vi "Initialize.vi"(8 "error in (no error)":errorcluster, 11 "S4ACS_GUI in":refnum<class "S4GUI.lvclass">) -> (0 "error out":errorcluster, 3 "S4ACS_GUI out":refnum<class "S4GUI.lvclass">)   [LabVIEW 2018, in "S4GUI.lvclass"]
uses:
  S4GUI.lvclass
  S4GUI.lvclass/S4GUI.ctl
  Publisher/Publisher.lvclass
  GSserver/GSserver.lvclass
  WeatherStation/WeatherStation.lvclass
  TelFocus/TelFocus.lvclass
  TCS/TCS.lvclass
  Instrument/Instrument.lvclass
  Acquisition/Acquisition.lvclass
  SyncBox/Sync Box.lvclass
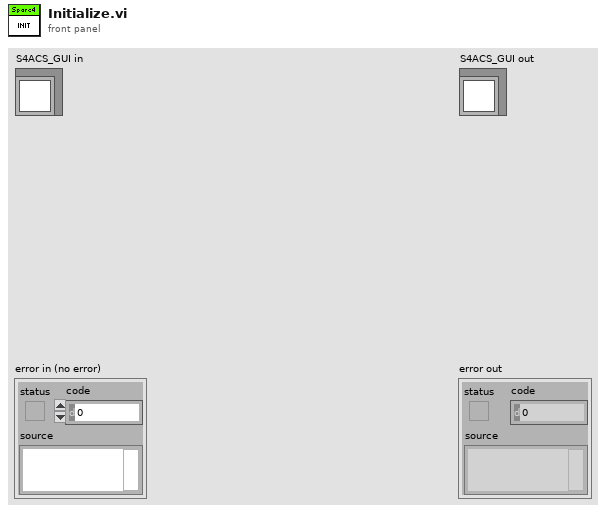
[diagram p1: front panel]
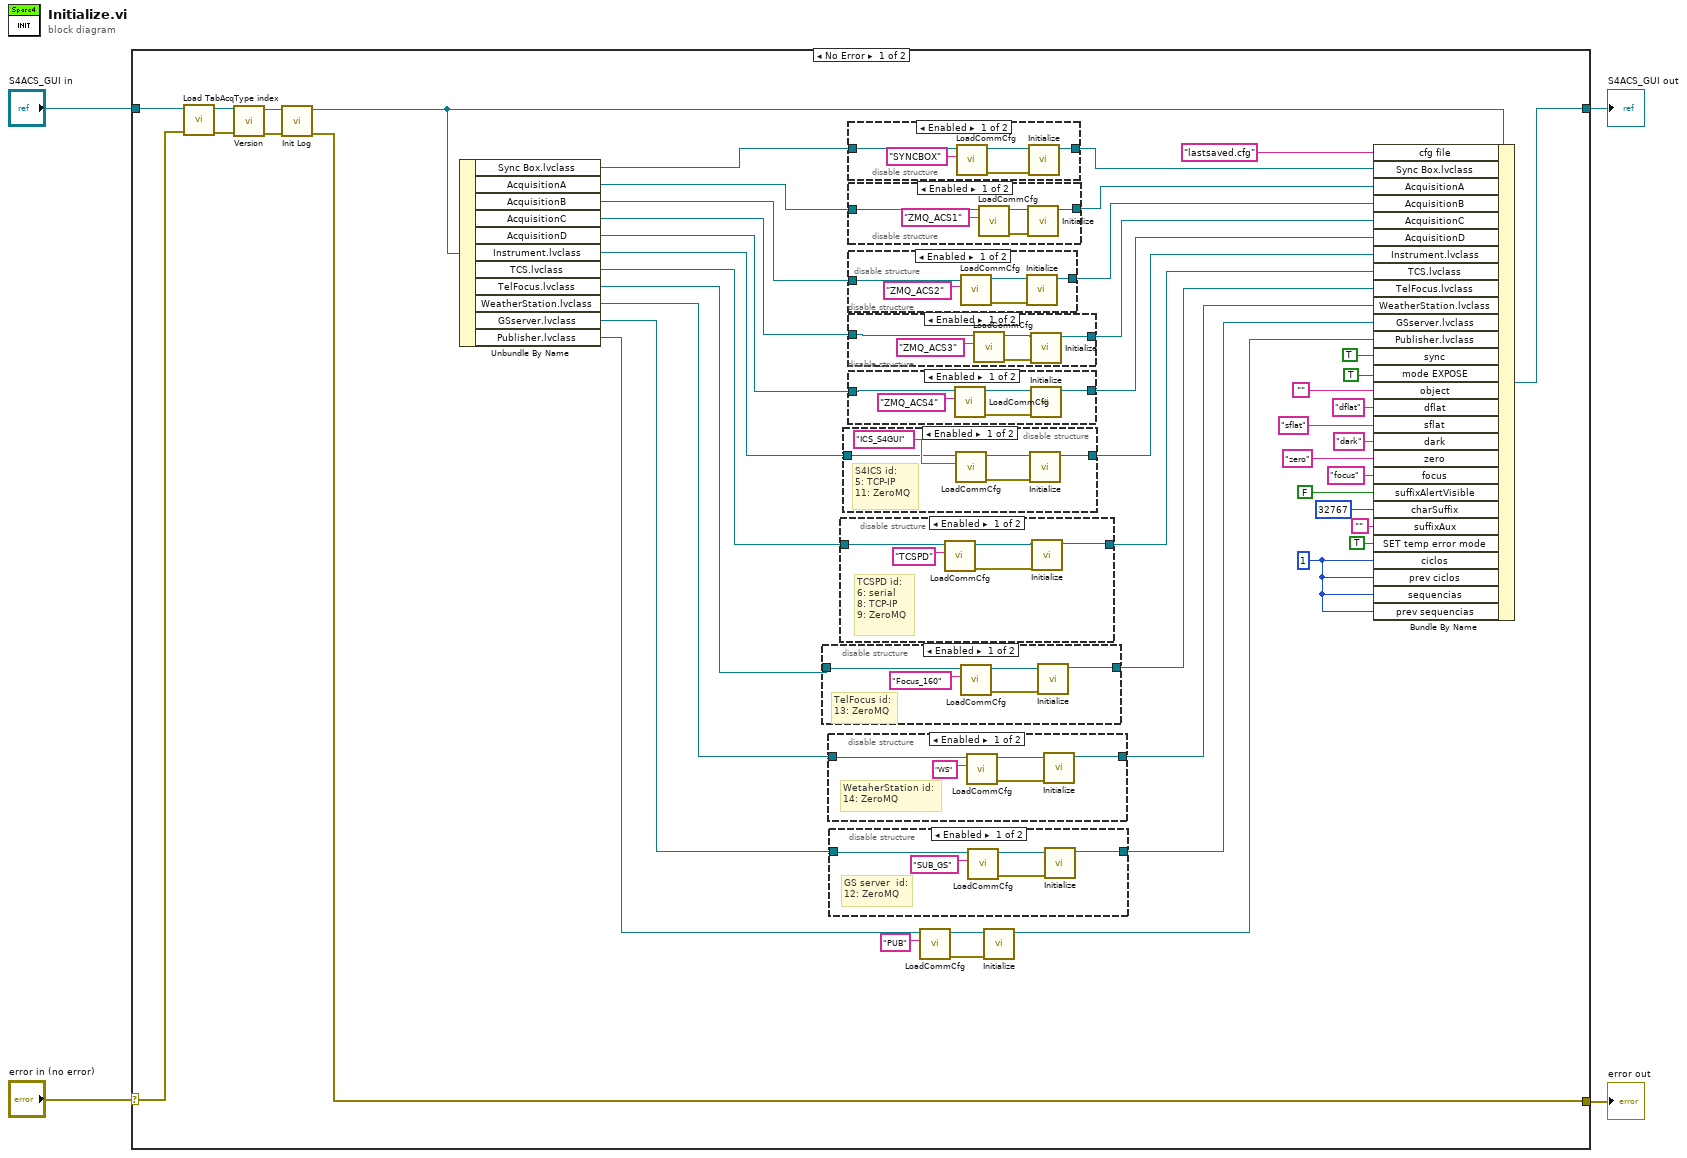
[diagram p0: block diagram]
diagram:
  n1 = case shown="No Error" "error in (no error)" {
    selector: "error in (no error)" -> [w20 w114]
    tunnel: [w23 w114] -> w3
    tunnel: [w31 w113] -> w1
    tunnel: "S4ACS_GUI in" -> [w18 w113]
    frame No Error {
      w5 = u32 1 ("ciclos")
      n2 = call-dynamic "Load TabAcqType index.vi"("error in (no error)"=w20, "S4GUI in"=w18) -> ("error out"=w19:errorcluster, "S4GUI out"=w17:refnum<class "S4GUI.lvclass">)  [unwired: 8 in]
      n3 = call-dynamic "Version.vi"("error in (no error)"=w19, "S4GUI in"=w17) -> ("error out"=w22:errorcluster, "S4GUI out"=w21:refnum<class "S4GUI.lvclass">)  [unwired: 8 in]
      n4 = call-dynamic "Init Log.vi"("error in (no error)"=w22, "S4GUI in"=w21) -> ("error out"=w23:errorcluster, "S4GUI out"=w37:refnum<class "S4GUI.lvclass">)  [unwired: 8 in]
      n5 = Unbundle By Name(w37) -> ("Sync Box.lvclass"=w43:refnum<class "Sync Box.lvclass">, "AcquisitionA"=w50:refnum<class "Acquisition.lvclass">, "AcquisitionB"=w49:refnum<class "Acquisition.lvclass">, "AcquisitionC"=w48:refnum<class "Acquisition.lvclass">, "AcquisitionD"=w47:refnum<class "Acquisition.lvclass">, "Instrument.lvclass"=w42:refnum<class "Instrument.lvclass">, "TCS.lvclass"=w39:refnum<class "TCS.lvclass">, "TelFocus.lvclass"=w36:refnum<class "TelFocus.lvclass">, "WeatherStation.lvclass"=w34:refnum<class "WeatherStation.lvclass">, "GSserver.lvclass"=w25:refnum<class "GSserver.lvclass">, "Publisher.lvclass"=w30:refnum<class "Publisher.lvclass">)
      n6 = disable-structure shown="Enabled" {
        disable-tunnel: w36 -> [w66 w70]
        disable-tunnel: [w65 w70] -> w35
        frame Enabled {
          # "TelFocus id:\n13: ZeroMQ"
          n7 = call-dynamic "LoadCommCfg.vi"("section (server name)"="Focus_160", "Server in"=w66) -> ("error out"=w67:errorcluster, "Server out"=w68:refnum<class "TelFocus.lvclass">)  [unwired: 8 in]
          n8 = call-dynamic "Initialize.vi"("error in (no error)"=w67, "TelFocus in"=w68) -> ("TelFocus out"=w65:refnum<class "TelFocus.lvclass">)  [unwired: 8 in, 1 out]
        }
        frame Disabled {
        }
      }
      n9 = disable-structure shown="Enabled" {
        disable-tunnel: w34 -> [w60 w64]
        disable-tunnel: [w59 w64] -> w32
        frame Enabled {
          # "WetaherStation id:\n14: ZeroMQ"
          n10 = call-dynamic "LoadCommCfg.vi"("section (server name)"="WS", "Server in"=w60) -> ("error out"=w61:errorcluster, "Server out"=w62:refnum<class "WeatherStation.lvclass">)  [unwired: 8 in]
          n11 = call-dynamic "Initialize.vi"("error in (no error)"=w61, "WeatherStation in"=w62) -> ("WeatherStation out"=w59:refnum<class "WeatherStation.lvclass">)  [unwired: 8 in, 1 out]
        }
        frame Disabled {
        }
      }
      n12 = disable-structure shown="Enabled" {
        disable-tunnel: w25 -> [w54 w58]
        disable-tunnel: [w53 w58] -> w24
        frame Enabled {
          # "GS server  id:\n12: ZeroMQ"
          n13 = call-dynamic "LoadCommCfg.vi"("section (server name)"="SUB_GS", "Server in"=w54) -> ("error out"=w55:errorcluster, "Server out"=w56:refnum<class "GSserver.lvclass">)  [unwired: 8 in]
          n14 = call-dynamic "Initialize.vi"("error in (no error)"=w55, "GSserver in"=w56) -> ("GSserver out"=w53:refnum<class "GSserver.lvclass">)  [unwired: 8 in, 1 out]
        }
        frame Disabled {
        }
      }
      n15 = disable-structure shown="Enabled" {
        disable-tunnel: w39 -> [w91 w94]
        disable-tunnel: [w93 w94] -> w38
        frame Enabled {
          # "TCSPD id:\n6: serial \n8: TCP-IP\n9: ZeroMQ"
          n16 = call-dynamic "LoadCommCfg.vi"("section (server name)"="TCSPD", "Server in"=w91) -> ("error out"=w89:errorcluster, "Server out"=w90:refnum<class "TCS.lvclass">)  [unwired: 8 in]
          n17 = call-dynamic "Initialize.vi"("error in (no error)"=w89, "TCS in"=w90) -> ("TCS out"=w93:refnum<class "TCS.lvclass">)  [unwired: 8 in, 1 out]
        }
        frame Disabled {
        }
      }
      n18 = disable-structure shown="Enabled" {
        disable-tunnel: w42 -> [w85 w88]
        disable-tunnel: [w87 w88] -> w41
        frame Enabled {
          # "S4ICS id:\n5: TCP-IP\n11: ZeroMQ"
          n19 = call-dynamic "LoadCommCfg.vi"("section (server name)"="ICS_S4GUI", "Server in"=w85) -> ("error out"=w83:errorcluster, "Server out"=w84:refnum<class "Instrument.lvclass">)  [unwired: 8 in]
          n20 = call-dynamic "Initialize.vi"("error in (no error)"=w83, "Instrument in"=w84) -> ("Instrument out"=w87:refnum<class "Instrument.lvclass">)  [unwired: 8 in, 1 out]
        }
        frame Disabled {
        }
      }
      n21 = disable-structure shown="Enabled" {
        disable-tunnel: [w111 w112] -> w44
        disable-tunnel: w43 -> [w110 w112]
        frame Enabled {
          n22 = call-dynamic "LoadCommCfg.vi"("section (server name)"="SYNCBOX", "Server in"=w110) -> ("error out"=w108:errorcluster, "Server out"=w109:refnum<class "Sync Box.lvclass">)  [unwired: 8 in]
          n23 = call-dynamic "Initialize.vi"("error in (no error)"=w108, "Sync Box in"=w109) -> ("Sync Box out"=w111:refnum<class "Sync Box.lvclass">)  [unwired: 8 in, 1 out]
        }
        frame Disabled {
        }
      }
      n24 = disable-structure shown="Enabled" {
        disable-tunnel: [w105 w106] -> w52
        disable-tunnel: w50 -> [w104 w106]
        frame Enabled {
          n25 = call-dynamic "LoadCommCfg.vi"("section (server name)"="ZMQ_ACS1", "Server in"=w104) -> ("error out"=w102:errorcluster, "Server out"=w103:refnum<class "Acquisition.lvclass">)  [unwired: 8 in]
          n26 = call-dynamic "Initialize.vi"("error in (no error)"=w102, "Acquisition in"=w103) -> ("Acquisition out"=w105:refnum<class "Acquisition.lvclass">)  [unwired: 8 in, 1 out]
        }
        frame Disabled {
        }
      }
      n27 = disable-structure shown="Enabled" {
        disable-tunnel: [w99 w100] -> w51
        disable-tunnel: w49 -> [w97 w100]
        frame Enabled {
          n28 = call-dynamic "LoadCommCfg.vi"("section (server name)"="ZMQ_ACS2", "Server in"=w97) -> ("error out"=w95:errorcluster, "Server out"=w96:refnum<class "Acquisition.lvclass">)  [unwired: 8 in]
          n29 = call-dynamic "Initialize.vi"("error in (no error)"=w95, "Acquisition in"=w96) -> ("Acquisition out"=w99:refnum<class "Acquisition.lvclass">)  [unwired: 8 in, 1 out]
        }
        frame Disabled {
        }
      }
      n30 = disable-structure shown="Enabled" {
        disable-tunnel: w48 -> [w79 w82]
        disable-tunnel: [w81 w82] -> w46
        frame Enabled {
          n31 = call-dynamic "LoadCommCfg.vi"("section (server name)"="ZMQ_ACS3", "Server in"=w79) -> ("error out"=w77:errorcluster, "Server out"=w78:refnum<class "Acquisition.lvclass">)  [unwired: 8 in]
          n32 = call-dynamic "Initialize.vi"("error in (no error)"=w77, "Acquisition in"=w78) -> ("Acquisition out"=w81:refnum<class "Acquisition.lvclass">)  [unwired: 8 in, 1 out]
        }
        frame Disabled {
        }
      }
      n33 = disable-structure shown="Enabled" {
        disable-tunnel: w47 -> [w73 w76]
        disable-tunnel: [w75 w76] -> w45
        frame Enabled {
          n34 = call-dynamic "LoadCommCfg.vi"("section (server name)"="ZMQ_ACS4", "Server in"=w73) -> ("error out"=w71:errorcluster, "Server out"=w72:refnum<class "Acquisition.lvclass">)  [unwired: 8 in]
          n35 = call-dynamic "Initialize.vi"("error in (no error)"=w71, "Acquisition in"=w72) -> ("Acquisition out"=w75:refnum<class "Acquisition.lvclass">)  [unwired: 8 in, 1 out]
        }
        frame Disabled {
        }
      }
      n36 = call-dynamic "LoadCommCfg.vi"("section (server name)"="PUB", "Client in"=w30) -> ("error out"=w28:errorcluster, "Client out"=w29:refnum<class "Publisher.lvclass">)  [unwired: 8 in]
      n37 = call-dynamic "Initialize.vi"("error in (no error)"=w28, "Client in"=w29) -> ("Client out"=w6:refnum<class "Publisher.lvclass">)  [unwired: 8 in, 1 out]
      n38 = Bundle By Name(cluster=w37, "cfg file"="lastsaved.cfg", "Sync Box.lvclass"=w44, "AcquisitionA"=w52, "AcquisitionB"=w51, "AcquisitionC"=w46, "AcquisitionD"=w45, "Instrument.lvclass"=w41, "TCS.lvclass"=w38, "TelFocus.lvclass"=w35, "WeatherStation.lvclass"=w32, "GSserver.lvclass"=w24, "Publisher.lvclass"=w6, "sync"=TRUE, "mode EXPOSE"=TRUE, "object"="" ("ClusterSuffix.object"), "dflat"="dflat" ("ClusterSuffix.dflat"), "sflat"="sflat" ("ClusterSuffix.sflat"), "dark"="dark" ("ClusterSuffix.dark"), "zero"="zero" ("ClusterSuffix.zero"), "focus"="focus" ("ClusterSuffix.focus"), "suffixAlertVisible"=FALSE, "charSuffix"=i16 32767 ("charKeyboard"), "suffixAux"="", "SET temp error mode"=TRUE, "ciclos"=w5, "prev ciclos"=w5, "sequencias"=w5, "prev sequencias"=w5) -> (w31:refnum<class "S4GUI.lvclass">)
    }
    frame Error {
    }
  }
  "error out" <- w3
  "S4ACS_GUI out" <- w1
